vi "Fpga-Get-Seconds.vi"(6 "upper":u16=7, 7 "lower":u16=2, 9 "Reset":bool, 10 "DataIn":u8, 11 "Index":u16) -> (2 "Valid":bool, 3 "UInt32":u32)   [LabVIEW 2016]
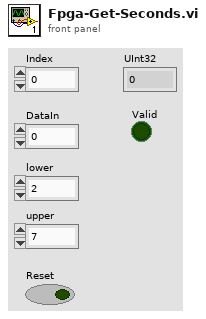
[diagram p1: front panel]
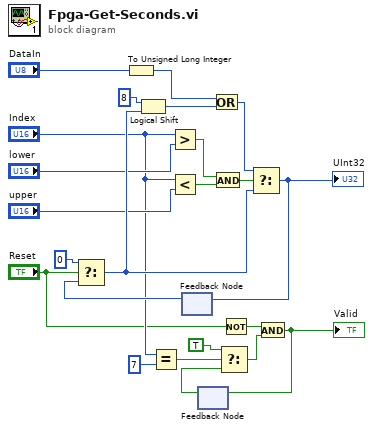
[diagram p0: block diagram]
diagram:
  n1 = To Unsigned Long Integer(number="DataIn") -> (unsigned 32bit integer=w14:u32)
  n2 = Equal?(x="Index", y=u16 7) -> (x = y?=w7:bool)
  n3 = Greater?(x="Index", y="lower") -> (0:w16:bool)
  n4 = Less?(x="Index", y="upper") -> (x < y?=w18:bool)
  n5 = feedback #1() -> (w21:u32)  [unwired: 1 in]
  n6 = Select(t=u32 0, s="Reset", f=w21) -> (s? t:f=w22:u32)
  n7 = Logical Shift(y=i16 8, x=w22) -> (x << y=w11:u32)
  n8 = feedback #2() -> (w5:bool)  [unwired: 1 in]
  n9 = Or(x=w14, y=w11) -> (x .or. y?=w12:u32)
  n10 = And(x=w16, y=w18) -> (x .and. y?=w15:bool)
  n11 = Select(t=TRUE, s=w7, f=w5) -> (s? t:f=w2:bool)
  n12 = Not(x="Reset") -> (.not. x?=w3:bool)
  n13 = Select(t=w12, s=w15, f=w22) -> (s? t:f=w20:u32)
  "UInt32" <- w20
  n14 = feedback-in #1(w20) -> ()
  n15 = And(x=w3, y=w2) -> (x .and. y?=w1:bool)
  "Valid" <- w1
  n16 = feedback-in #2(w1) -> ()
